vi "Initialize.vi"(8 "error in (no error)":errorcluster, 9 "Data Cluster (for Headers)":variant, 10 "TableLogger Config":T1, 11 "object in":refnum<class "TableLogger_CSV_Actor.lvclass">) -> (0 "error out":errorcluster, 3 "object out":refnum<class "TableLogger_CSV_Actor.lvclass">)   [LabVIEW 2014, in "TableLogger_CSV_Actor.lvlib" / "TableLogger_CSV_Actor.lvclass"]
uses:
  TableLogger_CSV_Actor.lvclass
  TableLogger_Actor/TableLoggerConfig.ctl
  TableLogger_Actor/TableLoggerTypes.ctl
  TableLogger_Actor/TableLoggerBackupConfig.ctl
  TableLogger_Actor/TableLogger_Actor/TableLogger_Actor.lvclass
  TableLogger_Actor/TableLogger_Actor.lvlib
panel:
  # "Connector Pane"
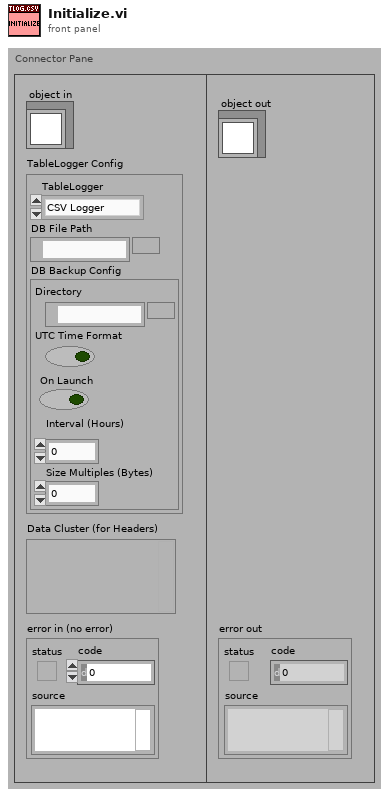
[diagram p1: front panel]
types:
  T1 = typedef "TableLogger_Actor.lvlib/TableLoggerConfig.ctl" = cluster{"TableLogger":T2, "DB File Path":path, "DB Backup Config":T3}
  T2 = typedef "TableLogger_Actor.lvlib/TableLoggerTypes.ctl" = enum16{"CSV Logger", "SQLite Logger"}
  T3 = typedef "TableLogger_Actor.lvlib/TableLoggerBackupConfig.ctl" = cluster{"Directory":path, "UTC Time Format":bool, "On Launch":bool, "Interval (Hours)":dbl, "Size Multiples (Bytes)":i32}
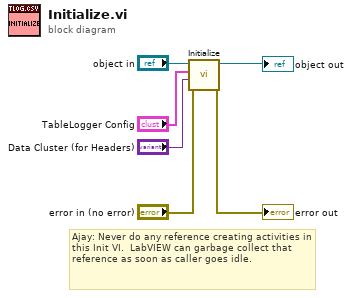
[diagram p0: block diagram]
diagram:
  # "Ajay: Never do any reference creating activities in this Init VI.  LabVIEW can garbage collect that reference as soon as caller goes idle."
  n1 = call-parent "Initialize.vi"("error in (no error)"="error in (no error)", "Data Cluster (for Headers)"="Data Cluster (for Headers)", "TableLogger Config"="TableLogger Config", "object in"="object in") -> ("error out"=→"error out":errorcluster, "object out"=→"object out":refnum<class "TableLogger_CSV_Actor.lvclass">)  [unwired: 6 in]
